vi "Strip JSON Path.vi"(11 "$Path":string) -> (1 "Child (B)":string, 2 "Base $Path (A)":string, 3 "$Path out":string)   [LabVIEW 2019, in "JSON-Schema.lvlib"]
uses:
  JSON-Schema.lvlib
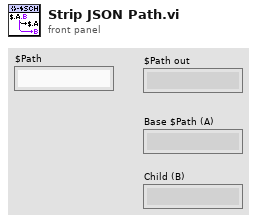
[diagram p1: front panel]
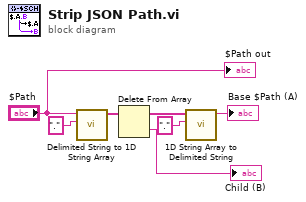
[diagram p0: block diagram]
diagram:
  n1 = call <vilib>:"Delimited String to 1D String Array.vi"("delimiter"=".", "delimited string"="$Path") -> ("string array"=w3:string[])  [unwired: 9 in]
  n2 = Delete From Array(array=w3) -> (deleted portion=→"Child (B)":string, array with subset deleted=w4:string[])  [unwired: 2 in]
  n3 = call <vilib>:"1D String Array to Delimited String.vi"("delimiter"=".", "string array"=w4) -> ("delimited string"=→"Base $Path (A)":string)  [unwired: 9 in]
  "$Path out" <- "$Path"
